vi "Write Subscriber List.vi"(8 "error in":errorcluster, 9 "Subscriber List":string[](array[string]), 10 "Topic Name":string, 11 "Broker in":refnum<class "Broker.lvclass">) -> (0 "error out":errorcluster, 3 "Broker out":refnum<class "Broker.lvclass">)   [LabVIEW 2014, in "Broker.lvclass"]
uses:
  Broker.lvclass
  Broker.lvclass/Broker.ctl
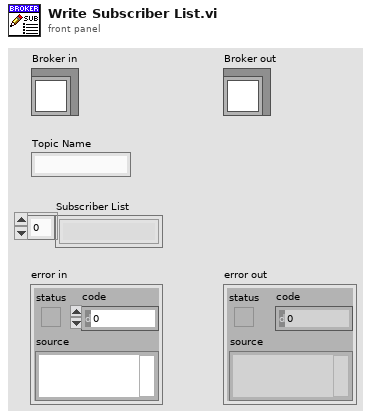
[diagram p1: front panel]
types:
  T1 = cluster{"Topic Name":string, "Subscriber List":string[]}[]
  T2 = cluster{"Topic Name":string, "Subscriber List":string[]}
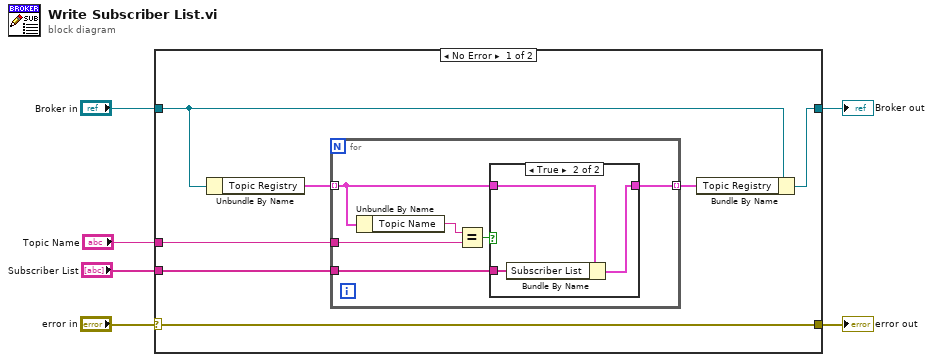
[diagram p0: block diagram]
diagram:
  n1 = case shown="No Error" "error in" {
    selector: "error in" -> [w13 w25]
    tunnel: [w13 w25] -> w5
    tunnel: [w8 w24] -> w3
    tunnel: "Broker in" -> [w9 w24]
    tunnel: "Topic Name" -> [w11 _]
    tunnel: "Subscriber List" -> [w10 _]
    frame No Error {
      n2 = Unbundle By Name(w9) -> ("Topic Registry"=w12:T1)
      n3 = for {
        tunnel: w12 -> [w19] mode=indexing
        tunnel: w11 -> [w16]
        tunnel: w10 -> [w18]
        tunnel: [w14] -> w7 mode=indexing
        n4 = Unbundle By Name(w19) -> ("Topic Name"=w17:string)
        n5 = Equal?(x=w17, y=w16) -> (x = y?=w15:bool)
        n6 = case shown="True" w15 {
          tunnel: w19 -> [w20 w23]
          tunnel: w18 -> [_ w22]
          tunnel: [w20 w21] -> w14
          frame False {
          }
          frame True {
            n7 = Bundle By Name(cluster=w23, "Subscriber List"=w22) -> (w21:T2)
          }
        }
      }
      n8 = Bundle By Name(cluster=w9, "Topic Registry"=w7) -> (w8:refnum<class "Broker.lvclass">)
    }
    frame Error {
    }
  }
  "error out" <- w5
  "Broker out" <- w3
